vi "TelemetryFieldToAddress.vi"(11 "TelemetryFields":T1=enum."InclinometerErrorCode") -> (3 "Address":u32)   [LabVIEW 2018]
uses:
  TelemetryFields.ctl
  <vilib>/Platform/TimedLoop/XDataNode/timing_clust.ctl
  <vilib>/Platform/TimedLoop/XDataNode/nitl_modes.ctl
  <vilib>/Platform/TimedLoop/XDataNode/wakeup.ctl
  <vilib>/rvi/Emulation/niFpgaSctlEmulationGetInTimedLoop.vi
  <vilib>/rvi/Emulation/niFpgaEmulationReportErrorSimple.vi
  <vilib>/rvi/Emulation/niFpgaGetClockAttributes.vi
  <vilib>/rvi/Emulation/niFpgaCriticalErrorInLSC.vi
  <vilib>/Platform/TimedLoop/XDataNode/XDataNode.xnode
  <vilib>/Platform/TimedLoop/XDataNode/XDNodeRunTimeDep.lvlib
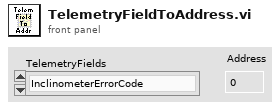
[diagram p1: front panel]
types:
  T1 = typedef "TelemetryFields.ctl" = enum16{"None", "InclinometerTxBytes", "InclinometerRxBytes", "InclinometerTxFrames", "InclinometerRxFrames", "InclinometerErrorTimestamp", "InclinometerErrorCode", "InclinometerSampleTimestamp", "InclinometerAngleRaw", "DisplacementTxBytes", "DisplacementRxBytes", "DisplacementTxFrames", "DisplacementRxFrames", "DisplacementErrorTimestamp", "DisplacementErrorCode", "DisplacementSampleTimestamp", "DisplacementRaw1", "DisplacementRaw2", "DisplacementRaw3", "DisplacementRaw4", "DisplacementRaw5", "DisplacementRaw6", "DisplacementRaw7", "DisplacementRaw8", "AccelerometerSampleCount", "AccelerometerSampleTimestamp", "AccelerometerRaw1", "AccelerometerRaw2", "AccelerometerRaw3", "AccelerometerRaw4", "AccelerometerRaw5", "AccelerometerRaw6", "AccelerometerRaw7", "AccelerometerRaw8", "GyroTxBytes", "GyroRxBytes", "GyroTxFrames", "GyroRxFrames", "GyroErrorTimestamp", "GyroErrorCode", "GyroSampleTimestamp", "GyroRawX", "GyroRawY", "GyroRawZ", "GyroStatus", "GyroSequenceNumber", "GyroTemperature", "GyroBITTimestamp", "GyroBIT0", "GyroBIT1", "GyroBIT2", "GyroBIT3", "GyroBIT4", "GyroBIT5", "GyroBIT6", "GyroBIT7", "DigitalInputSampleCount", "DigitalInputTimestamp", "DigitalInputStates", "DigitalOutputSampleCount", "DigitalOutputTimestamp", "DigitalOutputStates", "PowerSupplySampleCount", "PowerSupplyTimestamp", "PowerSupplyStates", "Modbus1ErrorFlags", "Modbus1TxByteCount", "Modbus1TxFrameCount", "Modbus1RxByteCount", "Modbus1RxFrameCount", "Modbus2ErrorFlags", "Modbus2TxByteCount", "Modbus2TxFrameCount", "Modbus2RxByteCount", "Modbus2RxFrameCount", "Modbus3ErrorFlags", "Modbus3TxByteCount", "Modbus3TxFrameCount", "Modbus3RxByteCount", "Modbus3RxFrameCount", "Modbus4ErrorFlags", "Modbus4TxByteCount", "Modbus4TxFrameCount", "Modbus4RxByteCount", "Modbus4RxFrameCount"}
  T2 = typedef "XDNodeRunTimeDep.lvlib/timing_clust.ctl" = cluster{"Expected End [f-1]":u64, "Actual End [f-1]":u64, "Finished Late? [f-1]":bool, "Expected End [i-1]":u64, "Actual End [i-1]":u64, "Finished Late? [i-1]":bool, "Expected Start [i]":u64, "Actual Start [i]":u64, "Expected Start [f]":u64, "Actual Start [f]":u64, "Source Name":string, "Structure Name":string, "Period":i64, "Deadline":i64, "Offset":i64, "Start":i64, "Priority":i32, "Timeout":i32, "Mode":T3, "Wakeup Reason":T4, "Error":errorcluster, "Source Type":string, "Secondary Source Type":string, "Global End Time":u64, "Global Start Time":u64, "Frame Duration":u64, "Iteration Duration":u64, "Assigned CPU":i32, "I/O Scan Engine Mode":u32}
  T3 = typedef "XDNodeRunTimeDep.lvlib/nitl_modes.ctl" = enum32{"No Change", "Process missed periods, maintain original phase", "Discard missed periods, maintain original phase", "Process missed periods, ignore original phase", "Discard missed periods, ignore original phase"}
  T4 = typedef "XDNodeRunTimeDep.lvlib/wakeup.ctl" = enum32{"Normal", "Aborted", "Asynchronous wakeup", "Timing source error", "Timed loop error", "Timeout"}
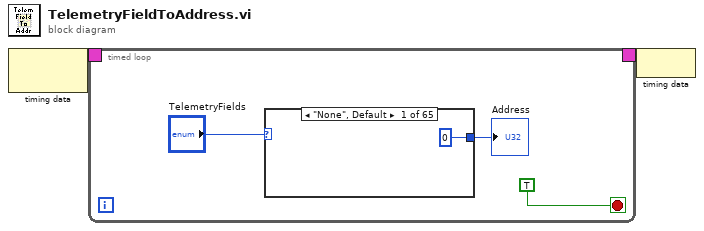
[diagram p0: block diagram]
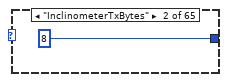
[diagram p2: hidden frame]
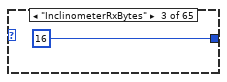
[diagram p3: hidden frame]
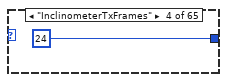
[diagram p4: hidden frame]
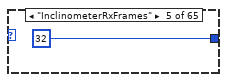
[diagram p5: hidden frame]
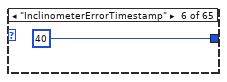
[diagram p6: hidden frame]
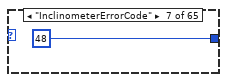
[diagram p7: hidden frame]
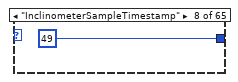
[diagram p8: hidden frame]
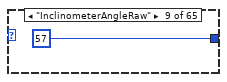
[diagram p9: hidden frame]
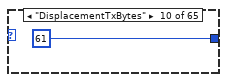
[diagram p10: hidden frame]
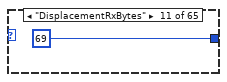
[diagram p11: hidden frame]
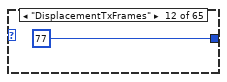
[diagram p12: hidden frame]
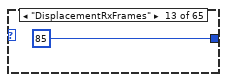
[diagram p13: hidden frame]
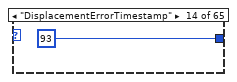
[diagram p14: hidden frame]
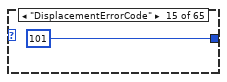
[diagram p15: hidden frame]
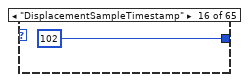
[diagram p16: hidden frame]
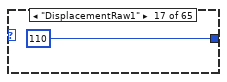
[diagram p17: hidden frame]
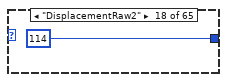
[diagram p18: hidden frame]
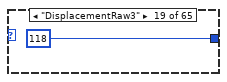
[diagram p19: hidden frame]
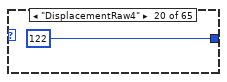
[diagram p20: hidden frame]
diagram:
  n1 = node-c288() -> (w2:T2)  [unwired: 1 in]
  n2 = timed-loop {
    timing: w2 -> [_]
    timing-out: [_] -> w1
    stop <- TRUE stop-if-true
    n3 = case shown="\"None\", Default" "TelemetryFields" {
      tunnel: [u32 0 ("Address") u32 8 ("Address") u32 16 ("Address") u32 24 ("Address") u32 32 ("Address") u32 40 ("Address") u32 48 ("Address") u32 49 ("Address") u32 57 ("Address") u32 61 ("Address") u32 69 ("Address") u32 77 ("Address") u32 85 ("Address") u32 93 ("Address") u32 101 ("Address") u32 102 ("Address") u32 110 ("Address") u32 114 ("Address") u32 118 ("Address") u32 122 ("Address") u32 126 ("Address") u32 130 ("Address") u32 134 ("Address") u32 138 ("Address") u32 142 ("Address") u32 150 ("Address") u32 158 ("Address") u32 162 ("Address") u32 166 ("Address") u32 170 ("Address") u32 174 ("Address") u32 178 ("Address") u32 182 ("Address") u32 186 ("Address") u32 190 ("Address") u32 198 ("Address") u32 206 ("Address") u32 214 ("Address") u32 222 ("Address") u32 230 ("Address") u32 231 ("Address") u32 239 ("Address") u32 243 ("Address") u32 247 ("Address") u32 251 ("Address") u32 252 ("Address") u32 253 ("Address") u32 255 ("Address") u32 263 ("Address") u32 264 ("Address") u32 265 ("Address") u32 266 ("Address") u32 267 ("Address") u32 268 ("Address") u32 269 ("Address") u32 270 ("Address") u32 271 ("Address") u32 279 ("Address") u32 287 ("Address") u32 289 ("Address") u32 297 ("Address") u32 305 ("Address") u32 306 ("Address") u32 314 ("Address") u32 322 ("Address")] -> w3
      frame "None", Default {
      }
      frame "InclinometerTxBytes" {
      }
      frame "InclinometerRxBytes" {
      }
      frame "InclinometerTxFrames" {
      }
      frame "InclinometerRxFrames" {
      }
      frame "InclinometerErrorTimestamp" {
      }
      frame "InclinometerErrorCode" {
      }
      frame "InclinometerSampleTimestamp" {
      }
      frame "InclinometerAngleRaw" {
      }
      frame "DisplacementTxBytes" {
      }
      frame "DisplacementRxBytes" {
      }
      frame "DisplacementTxFrames" {
      }
      frame "DisplacementRxFrames" {
      }
      frame "DisplacementErrorTimestamp" {
      }
      frame "DisplacementErrorCode" {
      }
      frame "DisplacementSampleTimestamp" {
      }
      frame "DisplacementRaw1" {
      }
      frame "DisplacementRaw2" {
      }
      frame "DisplacementRaw3" {
      }
      frame "DisplacementRaw4" {
      }
      frame "DisplacementRaw5" {
      }
      frame "DisplacementRaw6" {
      }
      frame "DisplacementRaw7" {
      }
      frame "DisplacementRaw8" {
      }
      frame "AccelerometerSampleCount" {
      }
      frame "AccelerometerSampleTimestamp" {
      }
      frame "AccelerometerRaw1" {
      }
      frame "AccelerometerRaw2" {
      }
      frame "AccelerometerRaw3" {
      }
      frame "AccelerometerRaw4" {
      }
      frame "AccelerometerRaw5" {
      }
      frame "AccelerometerRaw6" {
      }
      frame "AccelerometerRaw7" {
      }
      frame "AccelerometerRaw8" {
      }
      frame "GyroTxBytes" {
      }
      frame "GyroRxBytes" {
      }
      frame "GyroTxFrames" {
      }
      frame "GyroRxFrames" {
      }
      frame "GyroErrorTimestamp" {
      }
      frame "GyroErrorCode" {
      }
      frame "GyroSampleTimestamp" {
      }
      frame "GyroRawX" {
      }
      frame "GyroRawY" {
      }
      frame "GyroRawZ" {
      }
      frame "GyroStatus" {
      }
      frame "GyroSequenceNumber" {
      }
      frame "GyroTemperature" {
      }
      frame "GyroBITTimestamp" {
      }
      frame "GyroBIT0" {
      }
      frame "GyroBIT1" {
      }
      frame "GyroBIT2" {
      }
      frame "GyroBIT3" {
      }
      frame "GyroBIT4" {
      }
      frame "GyroBIT5" {
      }
      frame "GyroBIT6" {
      }
      frame "GyroBIT7" {
      }
      frame "DigitalInputSampleCount" {
      }
      frame "DigitalInputTimestamp" {
      }
      frame "DigitalInputStates" {
      }
      frame "DigitalOutputSampleCount" {
      }
      frame "DigitalOutputTimestamp" {
      }
      frame "DigitalOutputStates" {
      }
      frame "PowerSupplySampleCount" {
      }
      frame "PowerSupplyTimestamp" {
      }
      frame "PowerSupplyStates" {
      }
    }
    "Address" <- w3
  }
  n4 = node-c288(w1) -> ()
